vi "MALT Update Counters.vi"(8 "error in":errorcluster, 9 "Counters":i32=33, 10 "Address":i32=3, 11 "FamilyCode":T1=enum."MALT132") -> (0 "error out":errorcluster)   [LabVIEW 2018, in "AltonTech MALT200817.lvlib"]
uses:
  AltonTech MALT200817.lvlib
  Private/Types/MALT CardTypes.ctl
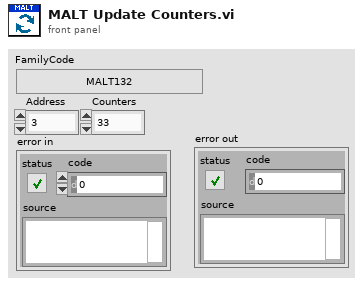
[diagram p1: front panel]
types:
  T1 = typedef "AltonTech MALT200817.lvlib/MALT CardTypes.ctl" = enum32{"-", "YAV90832", "YAV904X8", "MALT132", "YAV91616", "YAV90PIN", "YAV90096", "YAV90HVT", "YAV90CLR", "YAV90128", "YAV90PNE", "YAVCANCON", "YAV91775", "YAV90XXX", "YAV90MMU", "H730050", "H710060", "H710061", "YAV90304", "MMI", "YAV90060", "MALT160T", "YAV90059", "Not Defined"}
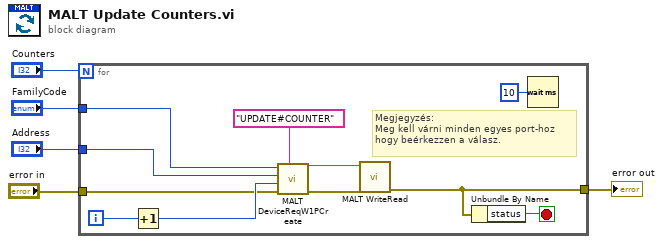
[diagram p0: block diagram]
diagram:
  n1 = for {
    N: "Counters" -> [_]
    tunnel: "error in" -> [w13]
    tunnel: [w8] -> w2
    tunnel: "FamilyCode" -> [w10]
    tunnel: "Address" -> [w9]
    i -> [w15]
    stop <- w7 stop-if-true
    # "Megjegyzés:\nMeg kell várni minden egyes port-hoz\nhogy beérkezzen a válasz."
    n2 = Increment(x=w15) -> (x+1=w14:i32)
    n3 = call "MALT DeviceReqW1PCreate.vi"("Cmd"="UPDATE#COUNTER", "error in"=w13, "Param1"=w14, "Address"=w9, "FamilyCode"=w10) -> ("error out"=w12:errorcluster, "Request"=w11:string)  [unwired: 5 in]
    n4 = call "MALT WriteRead.vi"("error in"=w12, "Request"=w11) -> ("error out"=w8:errorcluster)  [unwired: 8 in, 1 out]
    n5 = Unbundle By Name(w8) -> ("status"=w7:bool)
    n6 = Wait (ms)(milliseconds to wait=u32 10) -> ()  [unwired: 1 out]
  }
  "error out" <- w2
